vi "Curve Length.vi"(0 "start":dbl format="%.2f", 1 "end":dbl=1.0 format="%.2f", 2 "formula":string) -> (3 "X Values":dbl[](array[numeric]) format="%.2f", 4 "Curve Length":dbl[](array[numeric]) format="%.2f", 5 "ticks":u32, 6 "error":i32)   [LabVIEW 2020, in "NI_Gmath.lvlib"]
doc: "Calculates the curve length of a 1D function between <B>start</B> and <B>end</B>."
uses:
  <vilib>/gmath/NI_Gmath.lvlib
panel:
  # "Example:\n\n start: 0.0\n end: 1.0\n formula: sin(t)"
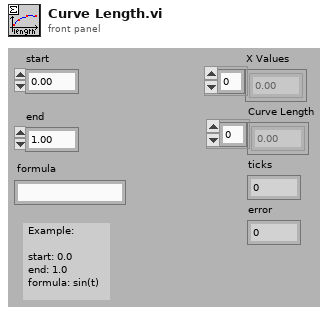
[diagram p1: front panel]
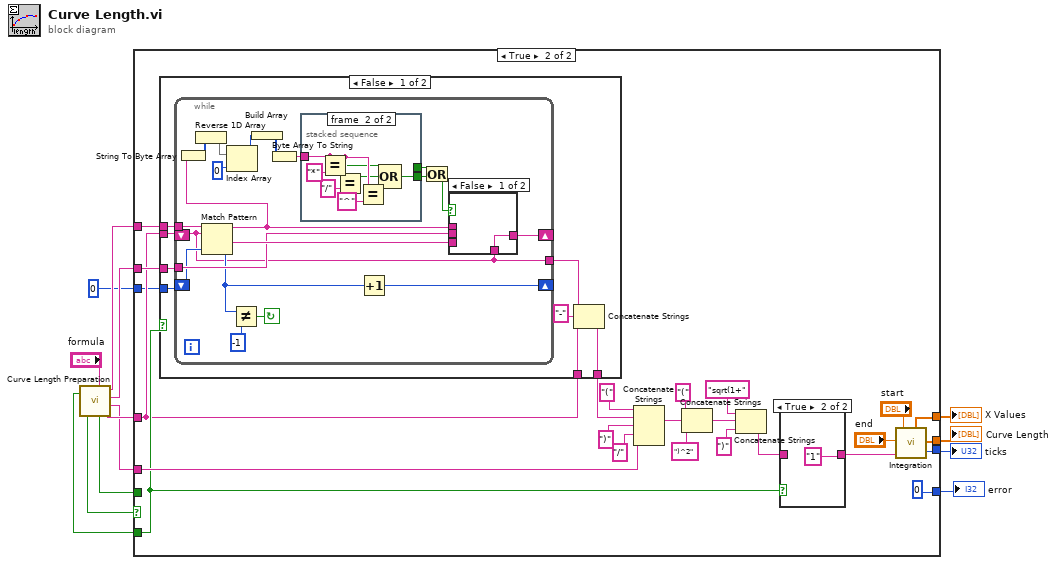
[diagram p0: block diagram]
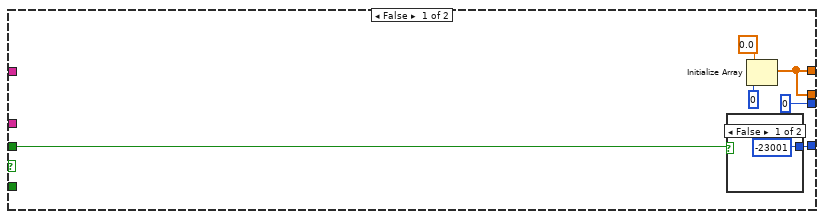
[diagram p2: hidden frame]
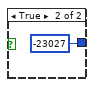
[diagram p3: hidden frame]
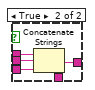
[diagram p5: hidden frame]
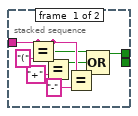
[diagram p6: hidden frame]
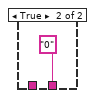
[diagram p7: hidden frame]
diagram:
  n1 = call <vilib>:"Curve Length Preparation.vi"("formula"="formula") -> ("correct number of variables"=w8:bool, "valid formula"=w13:bool, "error"=w9:bool, "string without spaces"=w6:string, "epsilon with brackets"=w5:string, "epsilon without brackets"=w2:string, "formula with brackets"=w3:string)
  n2 = case shown="True" w13 {
    tunnel: w3 -> [_ w23]
    tunnel: w2 -> [_ w33]
    tunnel: [u32 0 w28] -> w12
    tunnel: [w16 w27] -> w11
    tunnel: [w14 0] -> w10
    tunnel: w9 -> [w15 _]
    tunnel: w6 -> [_ w32]
    tunnel: w5 -> [_ w31]
    tunnel: w8 -> [_ w29]
    tunnel: [w16 w26] -> w7
    tunnel: 0 -> [_ w22]
    frame False {
      n3 = case shown="False" w15 {
        tunnel: [-23001 -23027] -> w14
        frame False {
        }
        frame True {
        }
      }
      n4 = Initialize Array(0.0, 0) -> (w16:dbl[])
    }
    frame True {
      n5 = case shown="False" w29 {
        tunnel: w31 -> [w55 _]
        tunnel: w23 -> [w54 _]
        tunnel: w32 -> [w53 _]
        tunnel: w23 -> [w51 _]
        tunnel: [w49 "0"] -> w24
        tunnel: w22 -> [w48 _]
        frame False {
          n6 = while {
            tunnel: [w56] -> w50
            tunnel: w55 -> [w73]
            shift-left: w48 -> [w69]
            shift-right: [w68] -> _
            tunnel: w53 -> [w75]
            shift-left: w54 -> [w56]
            shift-right: [w67] -> _
            stop <- w71 continue-if-true
            n7 = Match Pattern(string=w56, regular expression=w75, offset (0)=w69) -> (before substring=w66:string, after substring=w74:string, offset past match=w70:i32)  [unwired: 1 out]
            n8 = String To Byte Array(string=w66) -> (unsigned byte array=w65:u8[])
            n9 = Reverse 1D Array(array=w65) -> (reversed array=w64:u8[])
            n10 = Index Array(array=w64, index=0) -> (element=w62:u8)
            n11 = Not Equal?(x=w70, y=-1) -> (x != y?=w71:bool)
            n12 = Build Array(w62) -> (w61:u8[])
            n13 = Byte Array To String(unsigned byte array=w61) -> (string=w60:string)
            n14 = stacked-sequence {
              tunnel: w60 -> [w87 w95]
              tunnel: [_ w89] -> w59
              tunnel: [w81 _] -> w58
              frame #0 {
                n15 = Equal?(x=w87, y="(") -> (x = y?=w84:bool)
                n16 = Equal?(x=w87, y="+") -> (x = y?=w83:bool)
                n17 = Equal?(x=w87, y="-") -> (x = y?=w82:bool)
                n18 = Compound Arithmetic op=OR(w84, w83, w82) -> (w81:bool)
              }
              frame #1 {
                n19 = Equal?(x=w95, y="*") -> (x = y?=w92:bool)
                n20 = Equal?(x=w95, y="/") -> (x = y?=w91:bool)
                n21 = Equal?(x=w95, y="^") -> (x = y?=w90:bool)
                n22 = Compound Arithmetic op=OR(w92, w91, w90) -> (w89:bool)
              }
            }
            n23 = Increment(x=w70) -> (x+1=w68:i32)
            n24 = Or(x=w58, y=w59) -> (x .or. y?=w57:bool)
            n25 = case shown="False" w57 {
              tunnel: w66 -> [_ w80]
              tunnel: [w76 w79] -> w67
              tunnel: w73 -> [_ w78]
              tunnel: w74 -> [_ w77]
              tunnel: w56 -> [w76 _]
              frame False {
              }
              frame True {
                n26 = Concatenate Strings(w80, w78, w77) -> (w79:string)
              }
            }
          }
          n27 = Concatenate Strings(w50, "-", w51) -> (w49:string)
        }
        frame True {
        }
      }
      n28 = Concatenate Strings("(", w24, ")", "/", w33) -> (w42:string)
      n29 = Concatenate Strings("(", w42, ")^2") -> (w38:string)
      n30 = Concatenate Strings("sqrt(1+", w38, ")") -> (w25:string)
      n31 = case shown="True" w29 {
        tunnel: w25 -> [w46 _]
        tunnel: [w46 "1"] -> w30
        frame False {
        }
        frame True {
        }
      }
      n32 = call <vilib>:"Integration.vi"("formula"=w30, "end"="end", "start"="start") -> ("ticks"=w28:u32, "Integral of Y"=w27:dbl[], "X Values"=w26:dbl[])  [unwired: 2 out]
    }
  }
  "error" <- w10
  "ticks" <- w12
  "X Values" <- w7
  "Curve Length" <- w11
